vi "ACDC_Config.vi"(8 "error in (no error)":errorcluster, 10 "Data Rate [S/s]":u32, 11 "Input Config Array":T1[](array[typedef])=[0, 0, 0, 0, 0, 0, 0, 0, 0, 0, 0, 0, 0, 0, 0, 0, 0, 0, 0, 0, 0, 0, 0, 0, 0, 0, 0, 0, 0, 0, 0, 0] items=["AC Coupled", "DC Coupled", "IEPE AC Coupled"]) -> (0 "error out":errorcluster)   [LabVIEW 2017, in "VDMS_VibAPI_8.lvlib"]
uses:
  <vilib>/addons/InsightCM/Devices/Shared/Cms/Fpga/AcquisitionFpgaTach/source/subVIs/VibAPI_8/VDMS_VibAPI_8.lvlib
  <vilib>/LabVIEW Targets/FPGA/cRIO/shared/nicrio_ModuleControls/nicrio_cRIO-9232_ConfigModeRing.ctl
  <vilib>/LabVIEW Targets/FPGA/cRIO/shared/nicrio_ModuleControls/nicrio_cRIO-9232_DataRatesRing2.ctl
  <vilib>/rvi/eio/common/nirviEmuTemplatePropertySet_errors.vi
  <vilib>/eio/EIOPropertyNode/EIOPropertyNode.xnode
  <vilib>/rvi/eio/common/nirviEmuTemplatePropertyGet_errors.vi
  <vilib>/rvi/eio/common/nirviEmuTemplatePropertyGet_noerrors.vi
  <vilib>/rvi/eio/common/nirviEmuTemplatePropertySet_noerrors.vi
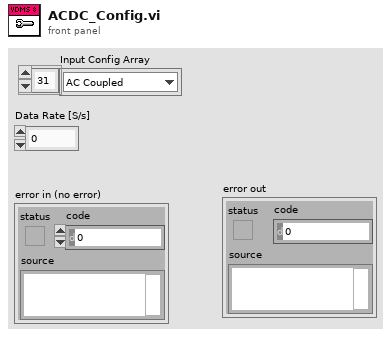
[diagram p1: front panel]
types:
  T1 = typedef "nicrio_cRIO-9232_ConfigModeRing.ctl" = u8
  T2 = typedef "nicrio_cRIO-9232_DataRatesRing2.ctl" = u8
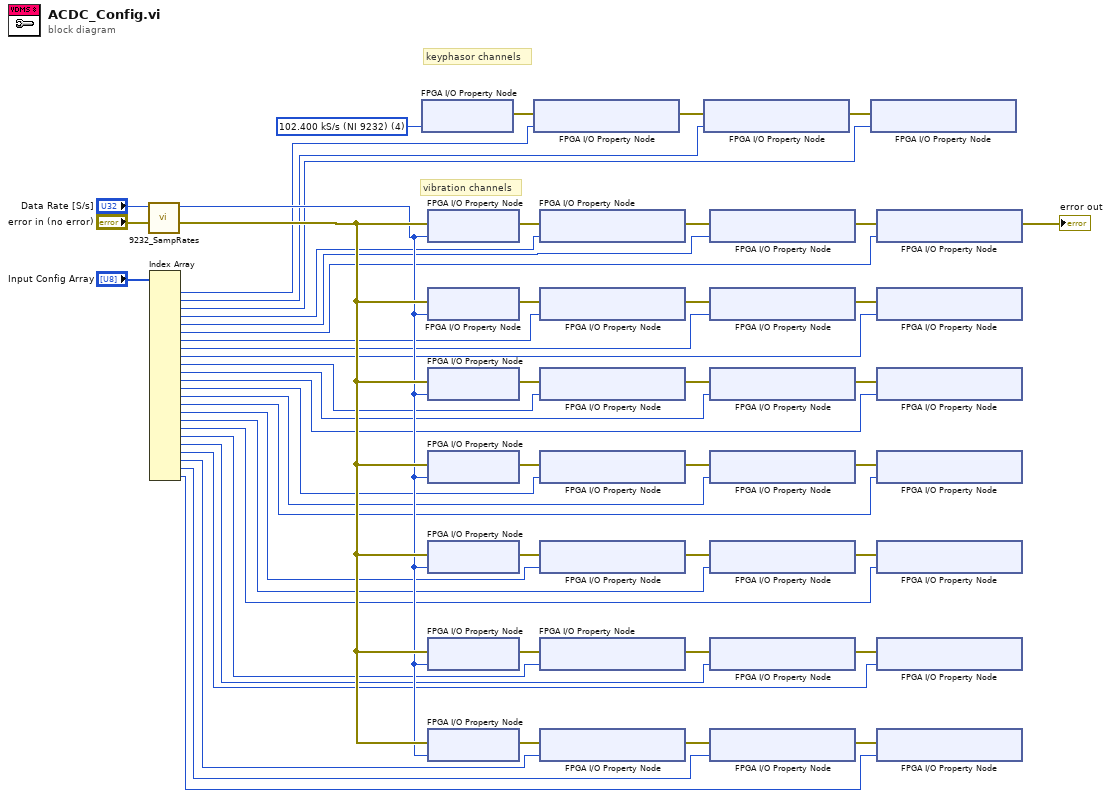
[diagram p0: block diagram]
diagram:
  w27 = T2 4 items=["102.400 kS/s (NI 9232)"=4, "51.200 kS/s (NI 9232)"=5, "34.133 kS/s (NI 9232)"=12, "25.600 kS/s (NI 9232)"=6, "20.480 kS/s (NI 9232)"=20, "17.067 kS/s (NI 9232)"=13, "14.629 kS/s (NI 9232)"=28, "12.800 kS/s (NI 9232)"=10, "11.378 kS/s (NI 9232)"=36, "10.240 kS/s (NI 9232)"=21, "9.309 kS/s (NI 9232)"=44, "8.533 kS/s (NI 9232)"=14, "7.877 kS/s (NI 9232)"=52, "7.314 kS/s (NI 9232)"=29, "6.827 kS/s (NI 9232)"=60, "6.400 kS/s (NI 9232)"=18, "6.024 kS/s (NI 9232)"=68, "5.689 kS/s (NI 9232)"=37, "5.389 kS/s (NI 9232)"=76, "5.120 kS/s (NI 9232)"=22, "4.876 kS/s (NI 9232)"=84, "4.655 kS/s (NI 9232)"=45, "4.452 kS/s (NI 9232)"=92, "4.267 kS/s (NI 9232)"=26, "4.096 kS/s (NI 9232)"=100, "3.938 kS/s (NI 9232)"=53, "3.657 kS/s (NI 9232)"=30, "3.413 kS/s (NI 9232)"=61, "3.200 kS/s (NI 9232)"=34, "3.012 kS/s (NI 9232)"=69, "2.844 kS/s (NI 9232)"=38, "2.695 kS/s (NI 9232)"=77, "2.560 kS/s (NI 9232)"=42, "2.438 kS/s (NI 9232)"=85, "2.327 kS/s (NI 9232)"=46, "2.226 kS/s (NI 9232)"=93, "2.133 kS/s (NI 9232)"=50, "2.048 kS/s (NI 9232)"=101, "1.969 kS/s (NI 9232)"=54, "1.829 kS/s (NI 9232)"=58, "1.707 kS/s (NI 9232)"=62, "1.600 kS/s (NI 9232)"=66, "1.506 kS/s (NI 9232)"=70, "1.422 kS/s (NI 9232)"=74, "1.347 kS/s (NI 9232)"=78, "1.280 kS/s (NI 9232)"=82, "1.219 kS/s (NI 9232)"=86, "1.164 kS/s (NI 9232)"=90, "1.113 kS/s (NI 9232)"=94, "1.067 kS/s (NI 9232)"=98, "1.024 kS/s (NI 9232)"=102, "0.985 kS/s (NI 9232)"=106] ("Data Rate")
  # "vibration channels"
  # "keyphasor channels"
  n1 = call <vilib>:"9232_SampRates.vi"("error in (no error)"="error in (no error)", "Data Rate [S/s]"="Data Rate [S/s]") -> ("error out"=w32:errorcluster, "Data Rate"=w26:T2)  [unwired: 8 in]
  n2 = Index Array(array="Input Config Array") -> (element #1=w24:T1, element #2=w23:T1, element #3=w22:T1, element #4=w21:T1, element #5=w20:T1, element #6=w19:T1, element #7=w18:T1, element #8=w17:T1, element #9=w16:T1, element #10=w15:T1, element #11=w14:T1, element #12=w13:T1, element #13=w12:T1, element #14=w11:T1, element #15=w10:T1, element #16=w9:T1, element #17=w8:T1, element #18=w7:T1, element #19=w6:T1, element #20=w5:T1, element #21=w4:T1, element #22=w3:T1, element #23=w2:T1, element #24=w1:T1)  [unwired: 24 in]
  n3 = xnode "FPGA I/O Property Node"("Data Rate"=w27) -> ("error out"=w30:errorcluster)  [unwired: 2 in, 1 out]
  n4 = xnode "FPGA I/O Property Node"("error in"=w32, "Data Rate"=w26) -> ("error out"=w51:errorcluster)  [unwired: 1 in, 1 out]
  n5 = xnode "FPGA I/O Property Node"("error in"=w32, "Data Rate"=w26) -> ("error out"=w33:errorcluster)  [unwired: 1 in, 1 out]
  n6 = xnode "FPGA I/O Property Node"("error in"=w32, "Data Rate"=w26) -> ("error out"=w46:errorcluster)  [unwired: 1 in, 1 out]
  n7 = xnode "FPGA I/O Property Node"("error in"=w32, "Data Rate"=w26) -> ("error out"=w45:errorcluster)  [unwired: 1 in, 1 out]
  n8 = xnode "FPGA I/O Property Node"("error in"=w32, "Data Rate"=w26) -> ("error out"=w40:errorcluster)  [unwired: 1 in, 1 out]
  n9 = xnode "FPGA I/O Property Node"("error in"=w32, "Data Rate"=w26) -> ("error out"=w39:errorcluster)  [unwired: 1 in, 1 out]
  n10 = xnode "FPGA I/O Property Node"("error in"=w32, "Data Rate"=w26) -> ("error out"=w34:errorcluster)  [unwired: 1 in, 1 out]
  n11 = xnode "FPGA I/O Property Node"("error in"=w30, "Input Configuration"=w24) -> ("error out"=w29:errorcluster)  [unwired: 1 in, 1 out]
  n12 = xnode "FPGA I/O Property Node"("error in"=w51, "Input Configuration"=w21) -> ("error out"=w52:errorcluster)  [unwired: 1 in, 1 out]
  n13 = xnode "FPGA I/O Property Node"("error in"=w33, "Input Configuration"=w18) -> ("error out"=w50:errorcluster)  [unwired: 1 in, 1 out]
  n14 = xnode "FPGA I/O Property Node"("error in"=w46, "Input Configuration"=w15) -> ("error out"=w47:errorcluster)  [unwired: 1 in, 1 out]
  n15 = xnode "FPGA I/O Property Node"("error in"=w45, "Input Configuration"=w12) -> ("error out"=w44:errorcluster)  [unwired: 1 in, 1 out]
  n16 = xnode "FPGA I/O Property Node"("error in"=w40, "Input Configuration"=w9) -> ("error out"=w41:errorcluster)  [unwired: 1 in, 1 out]
  n17 = xnode "FPGA I/O Property Node"("error in"=w39, "Input Configuration"=w6) -> ("error out"=w38:errorcluster)  [unwired: 1 in, 1 out]
  n18 = xnode "FPGA I/O Property Node"("error in"=w34, "Input Configuration"=w3) -> ("error out"=w35:errorcluster)  [unwired: 1 in, 1 out]
  n19 = xnode "FPGA I/O Property Node"("error in"=w29, "Input Configuration"=w23) -> ("error out"=w28:errorcluster)  [unwired: 1 in, 1 out]
  n20 = xnode "FPGA I/O Property Node"("error in"=w52, "Input Configuration"=w20) -> ("error out"=w53:errorcluster)  [unwired: 1 in, 1 out]
  n21 = xnode "FPGA I/O Property Node"("error in"=w50, "Input Configuration"=w17) -> ("error out"=w49:errorcluster)  [unwired: 1 in, 1 out]
  n22 = xnode "FPGA I/O Property Node"("error in"=w47, "Input Configuration"=w14) -> ("error out"=w48:errorcluster)  [unwired: 1 in, 1 out]
  n23 = xnode "FPGA I/O Property Node"("error in"=w44, "Input Configuration"=w11) -> ("error out"=w43:errorcluster)  [unwired: 1 in, 1 out]
  n24 = xnode "FPGA I/O Property Node"("error in"=w41, "Input Configuration"=w8) -> ("error out"=w42:errorcluster)  [unwired: 1 in, 1 out]
  n25 = xnode "FPGA I/O Property Node"("error in"=w38, "Input Configuration"=w5) -> ("error out"=w37:errorcluster)  [unwired: 1 in, 1 out]
  n26 = xnode "FPGA I/O Property Node"("error in"=w35, "Input Configuration"=w2) -> ("error out"=w36:errorcluster)  [unwired: 1 in, 1 out]
  n27 = xnode "FPGA I/O Property Node"("error in"=w28, "Input Configuration"=w22) -> ()  [unwired: 1 in, 2 out]
  n28 = xnode "FPGA I/O Property Node"("error in"=w53, "Input Configuration"=w19) -> ("error out"=→"error out":errorcluster)  [unwired: 1 in, 1 out]
  n29 = xnode "FPGA I/O Property Node"("error in"=w49, "Input Configuration"=w16) -> ()  [unwired: 1 in, 2 out]
  n30 = xnode "FPGA I/O Property Node"("error in"=w48, "Input Configuration"=w13) -> ()  [unwired: 1 in, 2 out]
  n31 = xnode "FPGA I/O Property Node"("error in"=w43, "Input Configuration"=w10) -> ()  [unwired: 1 in, 2 out]
  n32 = xnode "FPGA I/O Property Node"("error in"=w42, "Input Configuration"=w7) -> ()  [unwired: 1 in, 2 out]
  n33 = xnode "FPGA I/O Property Node"("error in"=w37, "Input Configuration"=w4) -> ()  [unwired: 1 in, 2 out]
  n34 = xnode "FPGA I/O Property Node"("error in"=w36, "Input Configuration"=w1) -> ()  [unwired: 1 in, 2 out]
